vi "uPython Comm.vi"() -> ()   [LabVIEW 2016]
uses:
  VIs/uPythonX/uPythonX.xctl
panel:
  in  "uPythonX":T1(xcontrol)
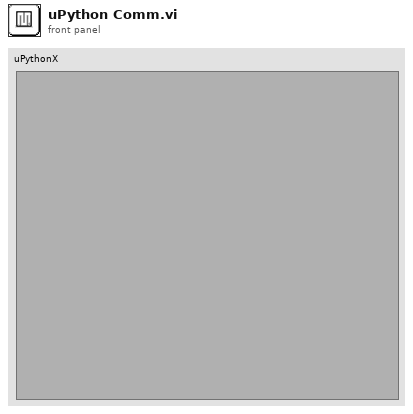
[diagram p1: front panel]
types:
  T1 = cluster{"VISA Refnum in":refnum<visa-resource-name>, "Python Code":string}
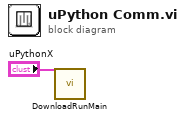
[diagram p0: block diagram]
diagram:
  n1 = call "DownloadRunMain.vi"("uPythonX"="uPythonX") -> ()  [unwired: 8 in, 3 out]
